vi "PCAN Get hardware name.vi"(7 "Language":T2 items=["System dependent", "Not available", "Not available", "Not available", "Not available", "Not available", "Not available", "Deutsch", "Not available", "English", "Español", "Not available", "Français", "Not available", "Not available", "Not available", "Italiano"], 8 "error in (no error)":errorcluster, 10 "Parameter":T3=enum."PCAN hardware name", 11 "Channel":T1) -> (0 "error out":errorcluster, 1 "Hardware name":string, 3 "Channel out":T1)   [LabVIEW 2020, in "PCANBasic.lvlib"]
doc: "PCAN_HARDWARE_NAME \n\nAccess: R\n\nDescription: This parameter is used to retrieve the name of the hardware represented by a PCAN channel. This is useful when an application wants to differentiate between several models of the same device, e.g. a PCAN-USB and a PCAN-USB Pro. \n\nPossible values: The value is a null-terminated string which contains the name of the hardware specified by the given PCAN channel. The length of this text will have a maximum length of 32 bytes (null-termination included). \n\nDefault value: NA. \n\nPCAN-Device: All PCAN devices (excluding PCAN_NONEBUS channel)."
uses:
  <vilib>/Sylvain.lib/user.lib/PCAN Basic/PCANBasic.lvlib
  <vilib>/Sylvain.lib/user.lib/PCAN Basic/Controls/Channel.ctl
  Controls/Parameter.ctl
  <vilib>/Sylvain.lib/user.lib/PCAN Basic/Controls/Error language selector.ctl
  PCANBasic.dll
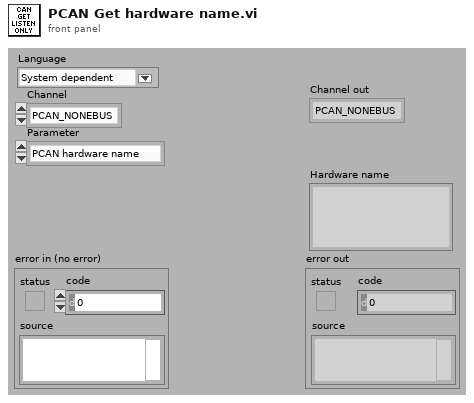
[diagram p1: front panel]
types:
  T1 = typedef "PCANBasic.lvlib/Channel.ctl" = enum16{"PCAN_NONEBUS", "not used1", "not used2", "not used3", "not used4", "not used5", "not used6", "not used7", "not used8", "not used9", "not used10", "not used11", "not used12", "not used13", "not used14", "not used15", "not used16", "not used17", "not used18", "not used19", "not used20", "not used21", "not used22", "not used23", "not used24", "not used25", "not used26", "not used27", "not used28", "not used29", "not used30", "not used31", "not used32", "PCAN_ISABUS1", "PCAN_ISABUS2", "PCAN_ISABUS3", "PCAN_ISABUS4", "PCAN_ISABUS5", "PCAN_ISABUS6", "PCAN_ISABUS7", "PCAN_ISABUS8", "not used41", "not used42", "not used43", "not used44", "not used45", "not used46", "not used47", "not used48", "PCAN_DNGBUS1", "not used50", "not used51", "not used52", "not used53", "not used54", "not used55", "not used56", "not used57", "not used58", "not used59", "not used60", "not used61", "not used62", "not used63", "not used64", "PCAN_PCIBUS1", "PCAN_PCIBUS2", "PCAN_PCIBUS3", "PCAN_PCIBUS4", "PCAN_PCIBUS5", "PCAN_PCIBUS6", "PCAN_PCIBUS7", "PCAN_PCIBUS8", "not used73", "not used74", "not used75", "not used76", "not used77", "not used78", "not used79", "not used80", "PCAN_USBBUS1", "PCAN_USBBUS2", "PCAN_USBBUS3", "PCAN_USBBUS4", "PCAN_USBBUS5", "PCAN_USBBUS6", "PCAN_USBBUS7", "PCAN_USBBUS8", "Not used89", "Not used90", "Not used91", "Not used92", "Not used93", "Not used94", "Not used95", "Not used96", "PCAN_PCCBUS1", "PCAN_PCCBUS2"}
  T2 = typedef "PCANBasic.lvlib/Error language selector.ctl" = u16
  T3 = typedef "PCANBasic.lvlib/Parameter.ctl" = enum16{"Not Available", "PCAN device number", "PCAN 5-volt power", "PCAN receive event", "PCAN message filter", "PCAN API version", "PCAN channel version", "PCAN bus-off auto reset", "PCAN listen-only", "PCAN log location", "PCAN log status", "PCAN log configure", "PCAN log text", "PCAN channel condition", "PCAN hardware name"}
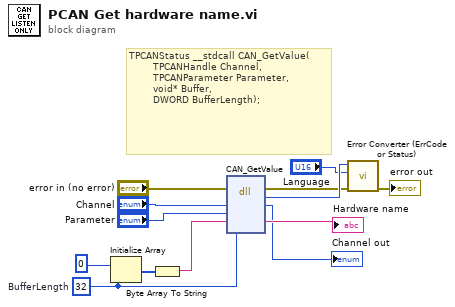
[diagram p0: block diagram]
diagram:
  w3 = u32 32  # BufferLength
  # "TPCANStatus __stdcall CAN_GetValue(\n        TPCANHandle Channel, \n        TPCANParameter Parameter,  \n        void* Buffer, \n        DWORD BufferLength);"
  n1 = Initialize Array(u8 0, w3) -> (w2:u8[])
  n2 = Byte Array To String(unsigned byte array=w2) -> (string=w1:string)
  n3 = dll-call lib="PCANBasic.*" fn="CAN_GetValue"(error in="error in (no error)", "Channel"="Channel", "Parameter"="Parameter", "Buffer"=w1, "BufferLength"=w3) -> (error out=w10:errorcluster, "return type"=w13:u32, "Channel"=→"Channel out":u8, "Buffer"=→"Hardware name":string)  [unwired: 4 in, 1 out]
  n4 = call <vilib>:"Error Converter (ErrCode or Status).vi"("error in (no error)"=w10, "Language"="Language", "error code"=w13) -> ("error out"=→"error out":errorcluster)  [unwired: 8 in]
